vi "Global 1.vi"() -> ()   [LabVIEW 2019]
panel:
  in  "tpg361_delay":u32=500
  in  "tpg361 COMPORT":refnum<visa-resource-name>
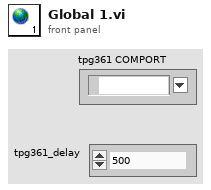
[diagram p1: front panel]
diagram:
